vi "myRIO_BRig_RT_dataBlock_init.vi"() -> (3 "output_dataBlock":u16[][](array[numeric]))   [LabVIEW 2014]
panel:
  # "0 - iBlock (Left)\n1 - nTrials (Left)\n2 - targetTrialsPerBlock (Left)\n3 - nRewards (Left)\n4 - Trials2Reward (Left)\n5 - BadTrialsPostReward (Left)\n\n6 - iBlock (Right)\n7 - nTrials (Right)\n8 - targetTrialsPerBlock (Right)\n9 - nRewards (Right)\n10 - Trials2Reward (Right)\n11 - BadTrialsPostReward (Right)"
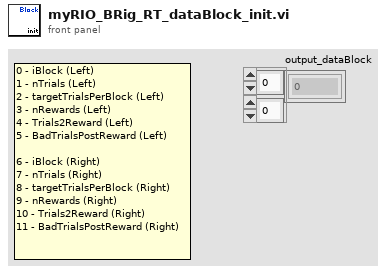
[diagram p1: front panel]
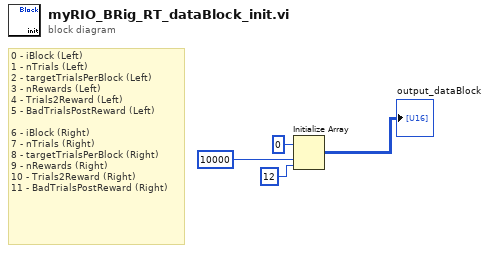
[diagram p0: block diagram]
diagram:
  # "0 - iBlock (Left)\n1 - nTrials (Left)\n2 - targetTrialsPerBlock (Left)\n3 - nRewards (Left)\n4 - Trials2Reward (Left)\n5 - BadTrialsPostReward (Left)\n\n6 - iBlock (Right)\n7 - nTrials (Right)\n8 - targetTrialsPerBlock (Right)\n9 - nRewards (Right)\n10 - Trials2Reward (Right)\n11 - BadTrialsPostReward (Right)"
  n1 = Initialize Array(u16 0 ("element"), 10000 ("dimension size"), 12 ("dimension size")) -> (→"output_dataBlock":u16[][])
